vi "oa_Check Spectrum Settings [OPS] (N Channels).vi"(6 "spectrum settings":cluster{"window type":u32, "block size":i32}={"window type"=1, "block size"=400} {"block size" min=2; "window type" items=["None"=0, "Hanning"=1, "Hamming"=2, "Blackman-Harris"=3, "Exact Blackman"=4, "Blackman"=5, "Flat Top"=6, "4 Term B-Harris"=7, "7 Term B-Harris"=8, "Low Sidelobe"=9, "Gaussian"=62]}, 8 "error in (no error)":errorcluster, 11 "resampled signals":cluster{"r0":dbl, "dr":dbl, "Y":dbl[]}[](array[cluster]) {"r0" format="%.2p"; "dr" format="%.2p"; "Y" format="%.2f"}) -> (0 "error out":errorcluster, 1 "parameter changed":bool, 3 "dup resampled signals":cluster{"r0":dbl, "dr":dbl, "Y":dbl[]}[](array[cluster]) {"r0" format="%.2p"; "dr" format="%.2p"; "Y" format="%.2f"})   [LabVIEW 2017, in "SoundVib_Resampling.lvlib"]
uses:
  <vilib>/addons/Sound and Vibration/Order Analysis/Resample Order Tracking/SoundVib_Resampling.lvlib
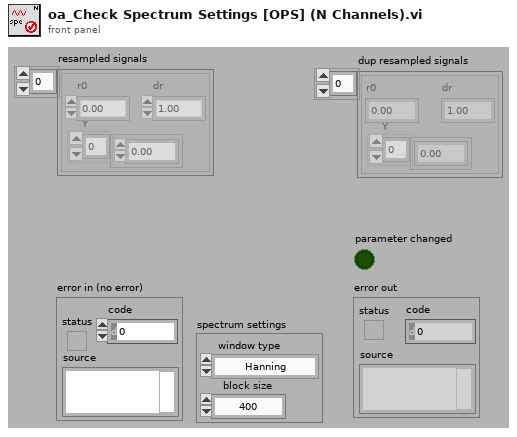
[diagram p1: front panel]
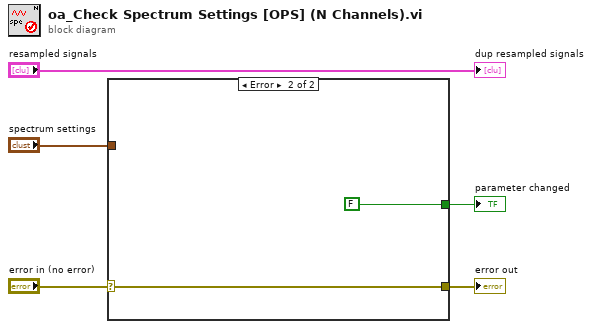
[diagram p0: block diagram]
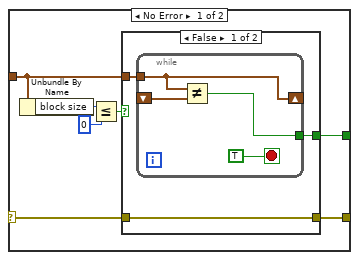
[diagram p2: hidden frame]
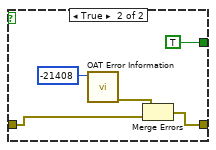
[diagram p3: hidden frame]
diagram:
  n1 = case shown="Error" "error in (no error)" {
    selector: "error in (no error)" -> [w6 w26]
    tunnel: [w7 w26] -> w4
    tunnel: "spectrum settings" -> [w11 _]
    tunnel: [w12 FALSE] -> w2
    frame No Error {
      n2 = Unbundle By Name(w11) -> ("block size"=w10:i32)
      n3 = Less Or Equal?(x=w10, y=0) -> (x <= y?=w8:bool)
      n4 = case shown="False" w8 {
        tunnel: [w15 TRUE] -> w12
        tunnel: w11 -> [w14 _]
        tunnel: [w13 w20] -> w7
        tunnel: w6 -> [w13 w21]
        frame False {
          n5 = while {
            tunnel: w14 -> [w17]
            shift-right: [w17] -> _
            shift-left: _ -> [w18]
            tunnel: [w16] -> w15
            stop <- TRUE stop-if-true
            n6 = Not Equal?(x=w17, y=w18) -> (x != y?=w16:bool)
          }
        }
        frame True {
          n7 = call <vilib>:"OAT Error Information.vi"("error code"=-21408) -> ("error out"=w22:errorcluster)  [unwired: 6 in]
          n8 = Merge Errors(w22, w21) -> (w20:errorcluster)
        }
      }
    }
    frame Error {
    }
  }
  "error out" <- w4
  "parameter changed" <- w2
  "dup resampled signals" <- "resampled signals"
